vi "Serial Input Channel Datapath.vi"(0 "arm":bool, 1 "reset":bool, 2 "resources":T16, 5 "stop":bool, 7 "timestamp counter value":T12, 9 "configuration":T1 {"channel acq config"."first packet data type select mask" format="%.0x"; "channel acq config"."last packet data type select mask" format="%.0x"}, 12 "ready for output":bool=TRUE) -> (4 "tagged llp packet":T3, 6 "end of data":bool, 8 "channel status":T13, 10 "tagged llp packet valid":bool, 14 "ready for arm":bool)   [LabVIEW 2020, in "GettingStarted_Acq_Tap_148X_FPGA.lvlib"]
uses:
  GettingStarted_Acq_Tap_148X_FPGA.lvlib
  Types/Serial Input Channel Resources.ctl
  <instrlib>/_niInstr/Memory/v1/FPGA/DRAM/niInstr Memory DRAM v1 FPGA.lvclass
  <instrlib>/FlexRIO/CSI-2/v2/FPGA/DRAM Manager/Private/DRAM Manager.ctl
  <instrlib>/FlexRIO/CSI-2/v2/FPGA/DRAM Manager/Private/Common/DRAM Manager Registers.ctl
  <instrlib>/FlexRIO/CSI-2/v2/FPGA/DRAM Manager/Private/Common/Handshake Registers.ctl
  <instrlib>/FlexRIO/CSI-2/v2/FPGA/DRAM Manager/Private/Common/DRAM Manager FIFOs.ctl
  <instrlib>/FlexRIO/CSI-2/v2/FPGA/DRAM Manager/Private/Common/Write Data FIFO Ref.ctl
  <instrlib>/FlexRIO/CSI-2/v2/FPGA/DRAM Manager/Private/Common/Read Request Metadata FIFO Ref.ctl
  <instrlib>/FlexRIO/CSI-2/v2/FPGA/DRAM Manager/Private/Common/Read Data FIFO Ref.ctl
  Types/Serial Input Channel IO.ctl
  Types/Serial Input Channel IO 32b.ctl
  Types/Serial Input Channel IO 64b.ctl
  Common/Types/I2C IO.ctl
  Types/Serial Input Channel Status.ctl
  <instrlib>/FlexRIO/CSI-2/v2/FPGA/Types/Channel-Based Acquisition Engine State.ctl
  Common/Types/DRAM Status.ctl
  <instrlib>/FlexRIO/CSI-2/v2/FPGA/Types/Timestamp Counter Value.ctl
  <instrlib>/FlexRIO/CSI-2/v2/FPGA/Types/Tagged LLP Packet.ctl
  <instrlib>/FlexRIO/CSI-2/v2/FPGA/Types/FPGA LLP Packet Tag.ctl
  <instrlib>/FlexRIO/CSI-2/v2/FPGA/Types/FPGA LLP Packet Timestamp.ctl
  <instrlib>/FlexRIO/CSI-2/v2/FPGA/Types/Timestamp ID.ctl
  <instrlib>/FlexRIO/CSI-2/v2/FPGA/Types/FPGA LLP Packet Size.ctl
  <instrlib>/FlexRIO/CSI-2/v2/FPGA/Types/LLP Packet.ctl
  <instrlib>/FlexRIO/CSI-2/v2/FPGA/Types/LLP Packet Header.ctl
  <instrlib>/FlexRIO/CSI-2/v2/FPGA/Types/LLP Packet Payload.ctl
  <instrlib>/FlexRIO/CSI-2/v2/FPGA/Types/LLP Packet Footer.ctl
  Types/Serial Input Channel Datapath Configuration.ctl
  <instrlib>/FlexRIO/CSI-2/v2/FPGA/Types/Channel-Based Acquistion Engine Configuration.ctl
  <instrlib>/FlexRIO/CSI-2/v2/FPGA/NI CSI-2 API FPGA v2.lvlib
  <instrlib>/_niInstr/Basic Elements/v1/FPGA/niInstr Basic Elements v1 FPGA.lvlib
  Common/GettingStarted_Common_148X_FPGA.lvlib
  <instrlib>/FlexRIO/CSI-2/v2/FPGA/DRAM Manager/DRAM Manager v2.lvlib
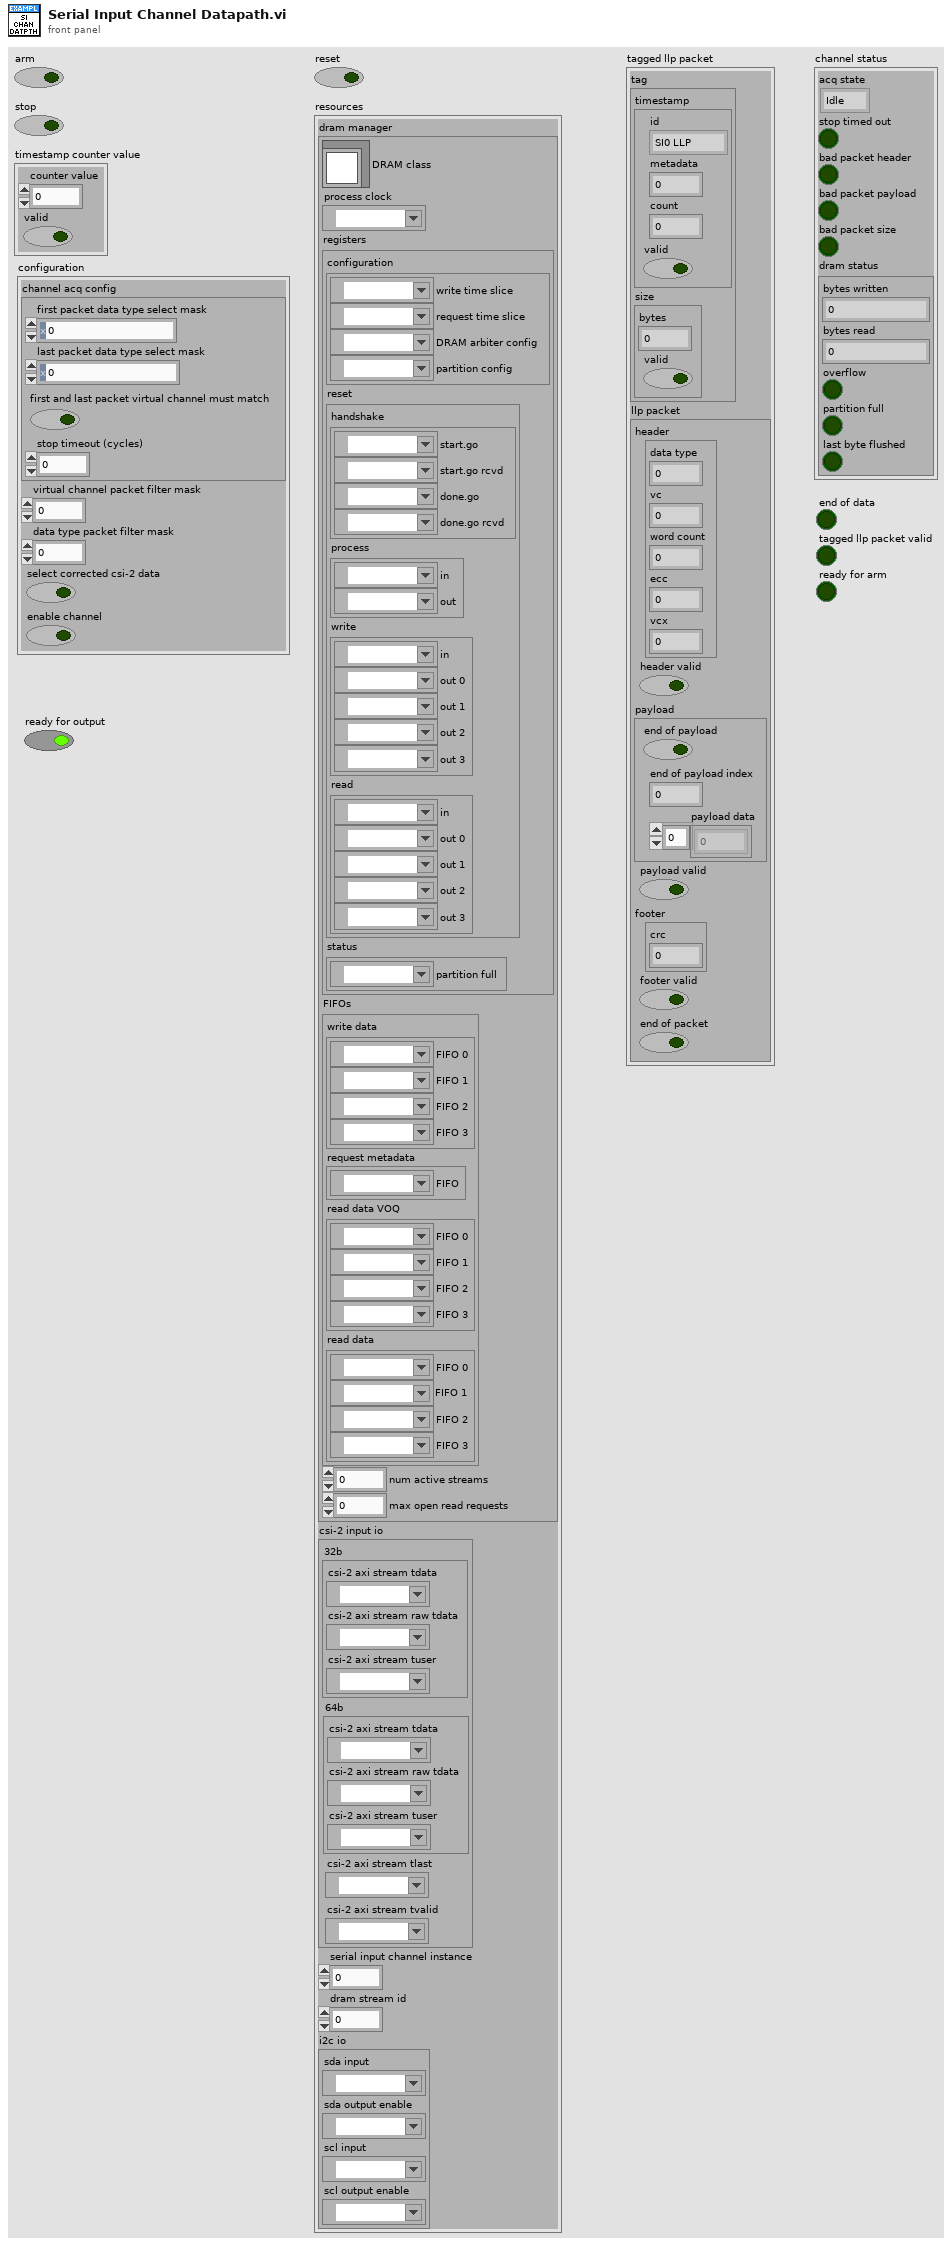
[diagram p1: front panel]
types:
  T1 = typedef "GettingStarted_Acq_Tap_148X_FPGA.lvlib/Serial Input Channel Datapath Configuration.ctl" = cluster{"channel acq config":T2, "virtual channel packet filter mask":u16, "data type packet filter mask":u64, "select corrected csi-2 data":bool, "enable channel":bool}
  T2 = typedef "NI CSI-2 API FPGA v2.lvlib/Channel-Based Acquistion Engine Configuration.ctl" = cluster{"stop timeout (cycles)":u32, "first packet data type select mask":u64, "last packet data type select mask":u64, "first and last packet virtual channel must match":bool}
  T3 = typedef "NI CSI-2 API FPGA v2.lvlib/Tagged LLP Packet.ctl" = cluster{"tag":T4, "llp packet":T8}
  T4 = typedef "NI CSI-2 API FPGA v2.lvlib/FPGA LLP Packet Tag.ctl" = cluster{"timestamp":T5, "size":T7}
  T5 = typedef "NI CSI-2 API FPGA v2.lvlib/FPGA LLP Packet Timestamp.ctl" = cluster{"valid":bool, "count":fxp<+,50,50>, "id":T6, "metadata":u8}
  T6 = typedef "NI CSI-2 API FPGA v2.lvlib/Timestamp ID.ctl" = enum8{"SI0 LLP", "SI1 LLP", "SI2 LLP", "SI3 LLP", "SI4 LLP", "SI5 LLP", "SI6 LLP", "SI7 LLP", "SO0 LLP", "SO1 LLP", "SO2 LLP", "SO3 LLP", "SO4 LLP", "SO5 LLP", "SO6 LLP", "SO7 LLP", "Ser0 GPIO Bank", "Ser1 GPIO Bank", "Ser2 GPIO Bank", "Ser3 GPIO Bank", "Ser4 GPIO Bank", "Ser5 GPIO Bank", "Ser6 GPIO Bank", "Ser7 GPIO Bank", "Des0 GPIO Bank", "Des1 GPIO Bank", "Des2 GPIO Bank", "Des3 GPIO Bank", "Des4 GPIO Bank", "Des5 GPIO Bank", "Des6 GPIO Bank", "Des7 GPIO Bank", "User0", "User1", "User2", "User3", "User4", "User5", "User6", "User7", "User8", "User9", "User10", "User11", "User12", "User13", "User14", "User15", "User16", "User17", "User18", "User19", "User20", "User21", "User22", "User23", "User24", "User25", "User26", "User27", "User28", "User29", "User30", "User31"}
  T7 = typedef "NI CSI-2 API FPGA v2.lvlib/FPGA LLP Packet Size.ctl" = cluster{"bytes":fxp<+,17,17>, "valid":bool}
  T8 = typedef "NI CSI-2 API FPGA v2.lvlib/LLP Packet.ctl" = cluster{"header":T9, "header valid":bool, "payload":T10, "payload valid":bool, "footer":T11, "footer valid":bool, "end of packet":bool}
  T9 = typedef "NI CSI-2 API FPGA v2.lvlib/LLP Packet Header.ctl" = cluster{"word count":u16, "ecc":fxp<+,6,6>, "vcx":fxp<+,2,2>, "data type":fxp<+,6,6>, "vc":fxp<+,2,2>}
  T10 = typedef "NI CSI-2 API FPGA v2.lvlib/LLP Packet Payload.ctl" = cluster{"end of payload":bool, "end of payload index":fxp<+,3,3>, "payload data":u8[]}
  T11 = typedef "NI CSI-2 API FPGA v2.lvlib/LLP Packet Footer.ctl" = cluster{"crc":u16}
  T12 = typedef "NI CSI-2 API FPGA v2.lvlib/Timestamp Counter Value.ctl" = cluster{"counter value":u64, "valid":bool}
  T13 = typedef "GettingStarted_Acq_Tap_148X_FPGA.lvlib/Serial Input Channel Status.ctl" = cluster{"acq state":T14, "stop timed out":bool, "bad packet header":bool, "bad packet payload":bool, "bad packet size":bool, "dram status":T15}
  T14 = typedef "NI CSI-2 API FPGA v2.lvlib/Channel-Based Acquisition Engine State.ctl" = enum8{"Idle", "Wait for First Packet Header", "Acquire", "Wait for Last Packet Header", "Wait for End of Last Packet"}
  T15 = typedef "GettingStarted_Common_148X_FPGA.lvlib/DRAM Status.ctl" = cluster{"bytes written":u64, "bytes read":u64, "overflow":bool, "partition full":bool, "last byte flushed":bool}
  T16 = typedef "GettingStarted_Acq_Tap_148X_FPGA.lvlib/Serial Input Channel Resources.ctl" = cluster{"dram manager":T17, "csi-2 input io":T24, "serial input channel instance":u8, "dram stream id":fxp<+,2,2>, "i2c io":T27}
  T17 = typedef "DRAM Manager v2.lvlib/DRAM Manager.ctl" = cluster{"DRAM class":refnum<class "niInstr Memory DRAM v1 FPGA.lvclass">, "process clock":refnum<k21>, "registers":T18, "FIFOs":T20, "num active streams":fxp<+,3,3>, "max open read requests":u16}
  T18 = typedef "DRAM Manager v2.lvlib/DRAM Manager Registers.ctl" = cluster{"configuration":cluster{"write time slice":refnum<k21>, "request time slice":refnum<k21>, "DRAM arbiter config":refnum<k21>, "partition config":refnum<k21>}, "reset":cluster{"handshake":T19, "process":cluster{"in":refnum<k21>, "out":refnum<k21>}, "write":cluster{"in":refnum<k21>, "out 0":refnum<k21>, "out 1":refnum<k21>, "out 2":refnum<k21>, "out 3":refnum<k21>}, "read":cluster{"in":refnum<k21>, "out 0":refnum<k21>, "out 1":refnum<k21>, "out 2":refnum<k21>, "out 3":refnum<k21>}}, "status":cluster{"partition full":refnum<k21>}}
  T19 = typedef "DRAM Manager v2.lvlib/Handshake Registers.ctl" = cluster{"start.go":refnum<k21>, "start.go rcvd":refnum<k21>, "done.go":refnum<k21>, "done.go rcvd":refnum<k21>}
  T20 = typedef "DRAM Manager v2.lvlib/DRAM Manager FIFOs.ctl" = cluster{"write data":cluster{"FIFO 0":T21, "FIFO 1":T21, "FIFO 2":T21, "FIFO 3":T21}, "request metadata":cluster{"FIFO":T22}, "read data VOQ":cluster{"FIFO 0":T23, "FIFO 1":T23, "FIFO 2":T23, "FIFO 3":T23}, "read data":cluster{"FIFO 0":T23, "FIFO 1":T23, "FIFO 2":T23, "FIFO 3":T23}}
  T21 = typedef "DRAM Manager v2.lvlib/Write Data FIFO Ref.ctl" = refnum<k21>
  T22 = typedef "DRAM Manager v2.lvlib/Read Request Metadata FIFO Ref.ctl" = refnum<k21>
  T23 = typedef "DRAM Manager v2.lvlib/Read Data FIFO Ref.ctl" = refnum<k21>
  T24 = typedef "GettingStarted_Acq_Tap_148X_FPGA.lvlib/Serial Input Channel IO.ctl" = cluster{"32b":T25, "64b":T26, "csi-2 axi stream tlast":refnum<k21>, "csi-2 axi stream tvalid":refnum<k21>}
  T25 = typedef "GettingStarted_Acq_Tap_148X_FPGA.lvlib/Serial Input Channel IO 32b.ctl" = cluster{"csi-2 axi stream tdata":refnum<k21>, "csi-2 axi stream raw tdata":refnum<k21>, "csi-2 axi stream tuser":refnum<k21>}
  T26 = typedef "GettingStarted_Acq_Tap_148X_FPGA.lvlib/Serial Input Channel IO 64b.ctl" = cluster{"csi-2 axi stream tdata":refnum<k21>, "csi-2 axi stream raw tdata":refnum<k21>, "csi-2 axi stream tuser":refnum<k21>}
  T27 = typedef "GettingStarted_Common_148X_FPGA.lvlib/I2C IO.ctl" = cluster{"sda input":refnum<k21>, "sda output enable":refnum<k21>, "scl input":refnum<k21>, "scl output enable":refnum<k21>}
  T28 = typedef "GettingStarted_Acq_Tap_148X_FPGA.lvlib/CSI-2 Status.ctl" = cluster{"start of transmission":bool, "header":bool, "header no error":bool, "header corrected error":bool, "header uncorrectable error":bool, " short packet":bool, "long packet header":bool, "end of transmission":bool, "good crc":bool, "bad crc":bool, "payload valids":fxp<+,4,4>, "checksum valids":fxp<+,4,4>, "filler valids":fxp<+,4,4>, "truncated packet error":bool, "upper payload valids":fxp<+,4,4>, "uppper checksum valids":fxp<+,4,4>, "upper filler valids":fxp<+,4,4>}
  T29 = typedef "NI CSI-2 API FPGA v2.lvlib/Timestamped LLP Packet.ctl" = cluster{"timestamp":T5, "llp packet":T8}
  T30 = typedef "NI CSI-2 API FPGA.lvlib/Tagged LLP Packet.ctl" = cluster{"tag":T31, "llp packet":T35}
  T31 = typedef "NI CSI-2 API FPGA.lvlib/FPGA LLP Packet Tag.ctl" = cluster{"timestamp":T32, "size":T34}
  T32 = typedef "NI CSI-2 API FPGA.lvlib/FPGA LLP Packet Timestamp.ctl" = cluster{"valid":bool, "count":fxp<+,50,50>, "id":T33, "metadata":u8}
  T33 = typedef "NI CSI-2 API FPGA.lvlib/Timestamp ID.ctl" = enum8{"SI0 LLP", "SI1 LLP", "SI2 LLP", "SI3 LLP", "SI4 LLP", "SI5 LLP", "SI6 LLP", "SI7 LLP", "SO0 LLP", "SO1 LLP", "SO2 LLP", "SO3 LLP", "SO4 LLP", "SO5 LLP", "SO6 LLP", "SO7 LLP", "Ser0 GPIO Bank", "Ser1 GPIO Bank", "Ser2 GPIO Bank", "Ser3 GPIO Bank", "Ser4 GPIO Bank", "Ser5 GPIO Bank", "Ser6 GPIO Bank", "Ser7 GPIO Bank", "Des0 GPIO Bank", "Des1 GPIO Bank", "Des2 GPIO Bank", "Des3 GPIO Bank", "Des4 GPIO Bank", "Des5 GPIO Bank", "Des6 GPIO Bank", "Des7 GPIO Bank", "User0", "User1", "User2", "User3", "User4", "User5", "User6", "User7", "User8", "User9", "User10", "User11", "User12", "User13", "User14", "User15", "User16", "User17", "User18", "User19", "User20", "User21", "User22", "User23", "User24", "User25", "User26", "User27", "User28", "User29", "User30", "User31"}
  T34 = typedef "NI CSI-2 API FPGA.lvlib/FPGA LLP Packet Size.ctl" = cluster{"bytes":fxp<+,17,17>, "valid":bool}
  T35 = typedef "NI CSI-2 API FPGA.lvlib/LLP Packet.ctl" = cluster{"header":T36, "header valid":bool, "payload":T37, "payload valid":bool, "footer":T38, "footer valid":bool, "end of packet":bool}
  T36 = typedef "NI CSI-2 API FPGA.lvlib/LLP Packet Header.ctl" = cluster{"word count":u16, "ecc":fxp<+,6,6>, "vcx":fxp<+,2,2>, "data type":fxp<+,6,6>, "vc":fxp<+,2,2>}
  T37 = typedef "NI CSI-2 API FPGA.lvlib/LLP Packet Payload.ctl" = cluster{"end of payload":bool, "end of payload index":fxp<+,2,2>, "payload data":u8[]}
  T38 = typedef "NI CSI-2 API FPGA.lvlib/LLP Packet Footer.ctl" = cluster{"crc":u16}
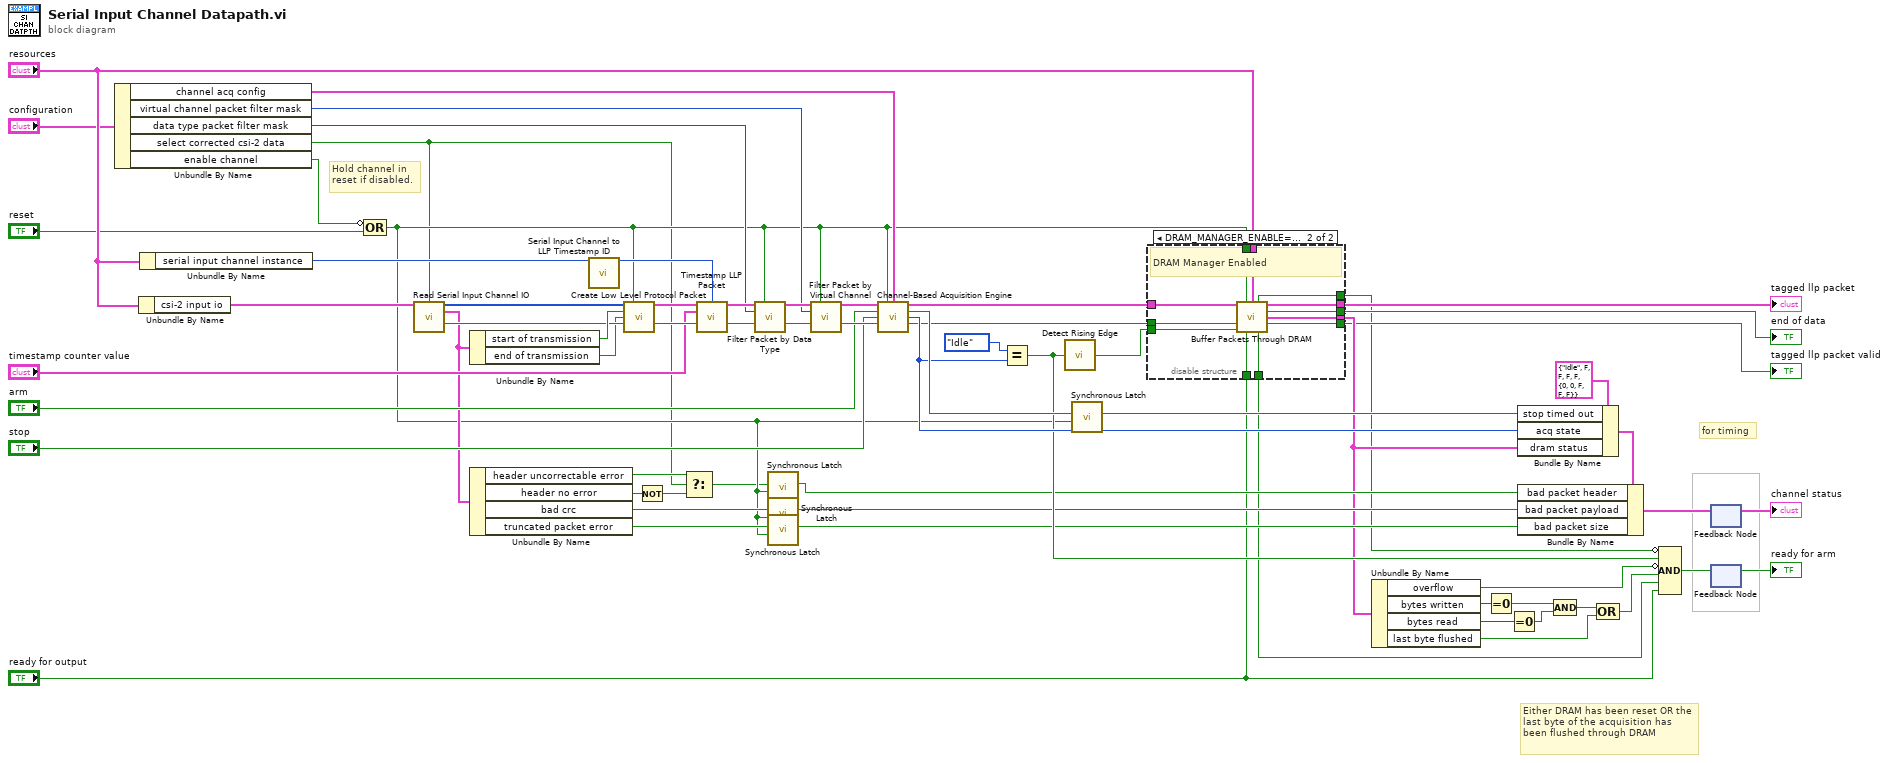
[diagram p0: block diagram]
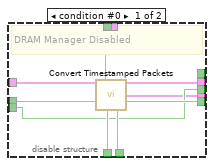
[diagram p2: hidden frame]
diagram:
  # "Either DRAM has been reset OR the last byte of the acquisition has been flushed through DRAM"
  # "for timing"
  # "Hold channel in \nreset if disabled."
  n1 = Unbundle By Name("configuration") -> ("channel acq config"=w50:T2, "virtual channel packet filter mask"=w51:u16, "data type packet filter mask"=w52:u64, "select corrected csi-2 data"=w13:bool, "enable channel"=w2:bool)
  n2 = Unbundle By Name("resources") -> ("csi-2 input io"=w45:T24)
  n3 = Unbundle By Name("resources") -> ("serial input channel instance"=w44:u8)
  n4 = Compound Arithmetic op=OR(invert w2, "reset") -> (w18:bool)
  n5 = call "Read Serial Input Channel IO.vi"("serial input channel io"=w45, "select corrected csi-2 data"=w13) -> ("csi-2 data"=w1:u8[], "csi-2 status"=w22:T28, "output valid"=w65:bool)  [unwired: 11 in]
  n6 = Unbundle By Name(w22) -> ("start of transmission"=w66:bool, "end of transmission"=w26:bool)
  n7 = Unbundle By Name(w22) -> ("header uncorrectable error"=w17:bool, "header no error"=w15:bool, "bad crc"=w21:bool, "truncated packet error"=w23:bool)
  n8 = call "Serial Input Channel to LLP Timestamp ID.vi"("serial input channel instance"=w44) -> ("llp timestamp id"=w47:T6)  [unwired: 14 in]
  n9 = call <instrlib>:"Create Low Level Protocol Packet.vi"("data"=w1, "reset"=w18, "start of transmission"=w66, "end of transmission"=w26, "input valid"=w65) -> ("llp packet"=w57:T8, "output valid"=w58:bool)  [unwired: 9 in]
  n10 = Not(x=w15) -> (.not. x?=w14:bool)
  n11 = Select(t=w17, s=w13, f=w14) -> (s? t:f=w16:bool)
  n12 = call <instrlib>:"Timestamp LLP Packet.vi"("llp packet in"=w57, "timestamp id"=w47, "timestamp counter value"="timestamp counter value", "input valid"=w58) -> ("timestamped llp packet"=w60:T29, "output valid"=w59:bool)  [unwired: 10 in]
  n13 = call <instrlib>:"Filter Packet by Data Type.vi"("timestamped llp packet"=w60, "reset"=w18, "packet data type filter mask"=w52, "input valid"=w59) -> ("filtered llp packet"=w62:T29, "output valid"=w64:bool)  [unwired: 9 in, 1 out]
  n14 = call <instrlib>:"Synchronous Latch.vi"("clear"=w18, "set"=w16) -> ("out"=w12:bool)  [unwired: 9 in]
  n15 = call <instrlib>:"Synchronous Latch.vi"("clear"=w18, "set"=w21) -> ("out"=w19:bool)  [unwired: 9 in]
  n16 = call <instrlib>:"Synchronous Latch.vi"("clear"=w18, "set"=w23) -> ("out"=w20:bool)  [unwired: 9 in]
  n17 = call <instrlib>:"Filter Packet by Virtual Channel.vi"("timestamped llp packet"=w62, "reset"=w18, "packet virtual channel filter mask"=w51, "input valid"=w64) -> ("filtered llp packet"=w61:T29, "output valid"=w63:bool)  [unwired: 9 in, 1 out]
  n18 = call <instrlib>:"Channel-Based Acquisition Engine.vi"("timestamped llp packet in"=w61, "reset"=w18, "configuration"=w50, "arm"="arm", "stop"="stop", "input valid"=w63) -> ("timestamped llp packet out"=w28:T29, "stop timed out"=w54:bool, "state"=w48:T14, "output valid"=w39:bool)  [unwired: 6 in]
  n19 = Equal?(x=Channel-Based_Acquisition_Engine_State."Idle" ("y"), y=w48) -> (x = y?=w30:bool)
  n20 = call <instrlib>:"Detect Rising Edge.vi"("signal"=w30) -> ("edge detected"=w37:bool)  [unwired: 14 in]
  n21 = call <instrlib>:"Synchronous Latch.vi"("clear"=w18, "set"=w54) -> ("out"=w49:bool)  [unwired: 9 in]
  n22 = disable-structure shown="DRAM_MANAGER_ENABLE==1, Default" {
    disable-tunnel: "resources" -> [_ w87]
    disable-tunnel: w39 -> [w73 w86]
    disable-tunnel: w37 -> [w68 w85]
    disable-tunnel: w28 -> [w74 w84]
    disable-tunnel: w18 -> [w72 w83]
    disable-tunnel: [w67 w82] -> w11
    disable-tunnel: [w75 w81] -> w10
    disable-tunnel: [w69 w80] -> w9
    disable-tunnel: [w68 w79] -> w8
    disable-tunnel: "ready for output" -> [w71 w78]
    disable-tunnel: [w70 w77] -> w6
    disable-tunnel: [_ w76] -> w5
    frame condition #0 {
      # "DRAM Manager Disabled"
      n23 = call "Convert Timestamped Packets.vi"("timestamped llp packet"=w74, "reset"=w72, "input valid"=w73, "ready for ouput"=w71) -> ("tagged llp packet"=w75:T30, "dram status"=w67:T15, "output valid"=w69:bool, "ready for input"=w70:bool)  [unwired: 8 in]
    }
    frame condition #1 (active) {
      # "DRAM Manager Enabled"
      n24 = call "Buffer Packets Through DRAM.vi"("timestamped llp packet"=w84, "reset"=w83, "resources"=w87, "input valid"=w86, "flush"=w85, "ready for output"=w78) -> ("in reset"=w76:bool, "tagged llp packet"=w81:T3, "end of data"=w79:bool, "dram status"=w82:T15, "output valid"=w80:bool, "ready for input"=w77:bool)  [unwired: 4 in]
    }
  }
  "tagged llp packet valid" <- w9
  "end of data" <- w8
  "tagged llp packet" <- w10
  n25 = Unbundle By Name(w11) -> ("overflow"=w38:bool, "bytes written"=w36:u64, "bytes read"=w35:u64, "last byte flushed"=w29:bool)
  n26 = Equal To 0?(x=w36) -> (x = 0?=w34:bool)
  n27 = Equal To 0?(x=w35) -> (x = 0?=w33:bool)
  n28 = Bundle By Name(cluster=T13 {"acq state"=enum."Idle", "stop timed out"=FALSE, "bad packet header"=FALSE, "bad packet payload"=FALSE, "bad packet size"=FALSE, "dram status"={"bytes written"=0, "bytes read"=0, "overflow"=FALSE, "partition full"=FALSE, "last byte flushed"=FALSE}} ("channel status"), "stop timed out"=w49, "acq state"=w48, "dram status"=w11) -> (w25:T13)
  n29 = Bundle By Name(cluster=w25, "bad packet header"=w12, "bad packet payload"=w19, "bad packet size"=w20) -> (w24:T13)
  n30 = Compound Arithmetic op=AND(w34, w33) -> (w32:bool)
  n31 = Compound Arithmetic op=OR(w32, w29) -> (w31:bool)
  n32 = Compound Arithmetic op=AND(invert w5, w30, invert w38, w31, w6, "ready for output") -> (w43:bool)
  n33 = feedback #1() -> (→"channel status":T13)  [unwired: 1 in]
  n34 = feedback-in #1(w24) -> ()
  n35 = feedback #2() -> (→"ready for arm":bool)  [unwired: 1 in]
  n36 = feedback-in #2(w43) -> ()
